vi "toindcluster.vi"(11 "data":T5) -> (1 "B[mT]":dbl, 2 "ROI":T3, 3 "Images":T1)   [LabVIEW 2013]
uses:
  dataTypdef.ctl
  <vilib>/vision/Image Controls.llb/IMAQ Image.ctl
  ROIStartfromCam_typdef.ctl
  classicROI_typDef.ctl
  analysis_data_typdef.ctl
  MagAnalysis_Online.lvclass
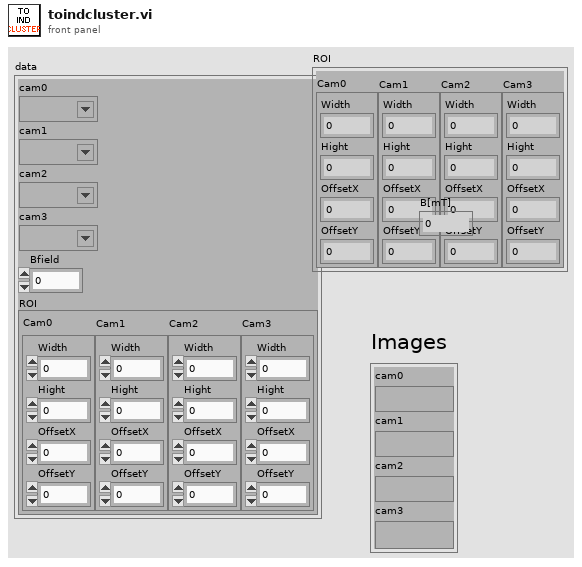
[diagram p1: front panel]
types:
  T1 = typedef "MagAnalysis_Online.lvclass/analysis_data_typdef.ctl" = cluster{"cam0":T2, "cam1":T2, "cam2":T2, "cam3":T2}
  T2 = typedef "IMAQ Image.ctl" = refnum<image>
  T3 = typedef "ROIStartfromCam_typdef.ctl" = cluster{"Cam0":T4, "Cam1":T4, "Cam2":T4, "Cam3":T4}
  T4 = typedef "classicROI_typDef.ctl" = cluster{"Width":dbl, "Hight":dbl, "OffsetX":dbl, "OffsetY":dbl}
  T5 = typedef "dataTypdef.ctl" = cluster{"cam0":T2, "cam1":T2, "cam2":T2, "cam3":T2, "Bfield":dbl, "ROI":T3}
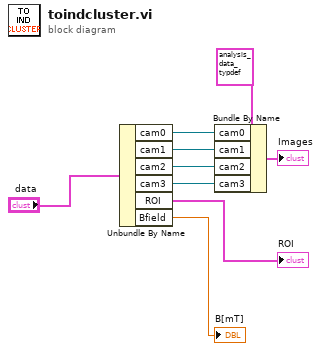
[diagram p0: block diagram]
diagram:
  n1 = Unbundle By Name("data") -> ("cam0"=w7:T2, "cam1"=w6:T2, "cam2"=w5:T2, "cam3"=w4:T2, "ROI"=→"ROI":T3, "Bfield"=→"B[mT]":dbl)
  n2 = Bundle By Name(cluster=T1 {"cam0"=refnum, "cam1"=refnum, "cam2"=refnum, "cam3"=refnum} ("Images 2"), "cam0"=w7, "cam1"=w6, "cam2"=w5, "cam3"=w4) -> (→"Images":T1)
